vi "Configure Clock Source.vi"(8 "error in (no error)":errorcluster, 10 "Source (0: Internal)":u16(ring) items=["Internal", "External"], 11 "VISA resource name":refnum<visa-resource-name>) -> (0 "error out":errorcluster, 2 "Error?":bool, 3 "VISA resource name out":refnum<visa-resource-name>)   [LabVIEW 2017, in "Siglent SDG 1000 5000 800 Series.lvlib"]
doc: "Selects the reference clock source/oscillator for signal generation.\n\nNote: This function is not available on models SDG805, SDG810, SDG830."
uses:
  <instrlib>/Siglent SDG 1000 5000 800 Series/Siglent SDG 1000 5000 800 Series.lvlib
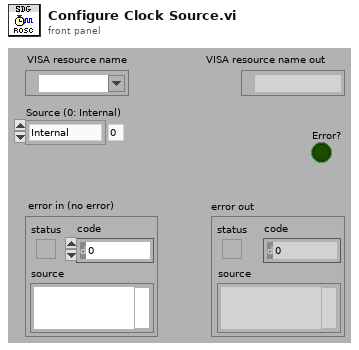
[diagram p1: front panel]
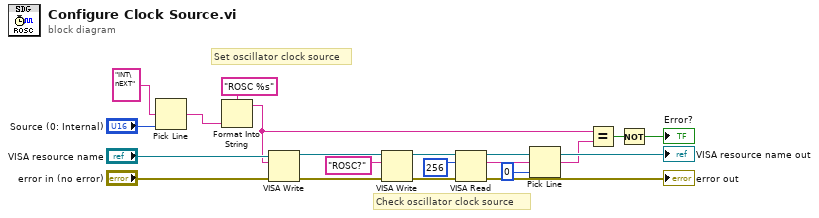
[diagram p0: block diagram]
diagram:
  # "Check oscillator clock source"
  # "Set oscillator clock source"
  n1 = Pick Line(multi-line string="INT\nEXT", line index="Source (0: Internal)") -> (output string=w15:string)  [unwired: 1 in]
  n2 = Format Into String(format string="ROSC %s", w15) -> (resulting string=w6:string)  [unwired: 2 in, 1 out]
  n3 = VISA Write(VISA resource name="VISA resource name", write buffer=w6, error in (no error)="error in (no error)") -> (VISA resource name out=w9:refnum<visa-resource-name>, error out=w10:errorcluster)  [unwired: 1 out]
  n4 = VISA Write(VISA resource name=w9, write buffer="ROSC?", error in (no error)=w10) -> (VISA resource name out=w8:refnum<visa-resource-name>, error out=w7:errorcluster)  [unwired: 1 out]
  n5 = VISA Read(VISA resource name=w8, byte count=u32 256, error in (no error)=w7) -> (VISA resource name out=→"VISA resource name out":refnum<visa-resource-name>, read buffer=w3:string, error out=→"error out":errorcluster)  [unwired: 1 out]
  n6 = Pick Line(multi-line string=w3, line index=0) -> (output string=w2:string)  [unwired: 1 in]
  n7 = Equal?(x=w6, y=w2) -> (x = y?=w5:bool)
  n8 = Not(x=w5) -> (.not. x?=→"Error?":bool)
